vi "Neighbors.vi"(7 "Position":T1, 11 "Team In":i32[][](array[numeric])) -> (2 "Neighbors":i32[](array[numeric]), 3 "Team":i32[][](array[numeric]))   [LabVIEW 2020, in "SquareBattle.lvlib" / "Map.lvclass"]
uses:
  Map.lvclass
  Position.ctl
  SquareBattle.lvlib
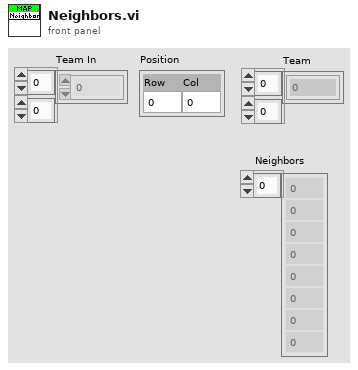
[diagram p1: front panel]
types:
  T1 = typedef "SquareBattle.lvlib/Position.ctl" = cluster{"Row":i32, "Col":i32}
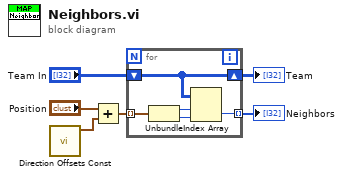
[diagram p0: block diagram]
diagram:
  n1 = call "Direction Offsets Const.vi"() -> ("Direction Offsets"=w1:T1[])  [unwired: 11 in]
  n2 = Add(x="Position", y=w1) -> (x+y=w3:T1[])
  n3 = for {
    shift-right: [w10] -> w5
    shift-left: "Team In" -> [w10]
    tunnel: w3 -> [w11] mode=indexing
    tunnel: [w7] -> w2 mode=indexing
    n4 = Unbundle(w11) -> ("Row"=w9:i32, "Col"=w8:i32)
    n5 = Index Array(array=w10, index (row)=w9, index (col)=w8) -> (element=w7:i32)
  }
  "Team" <- w5
  "Neighbors" <- w2
